vi "VIPM Project Parser_To String.vi"(11 "External Target Element":T1) -> (3 "Dependencies":string[](array[string]))   [LabVIEW 2019]
uses:
  Build/Project.Dependencies Finder.lvlibp/Ctl/Ctl_Dependency Element.ctl
  Build/Project.Dependencies Finder.lvlibp
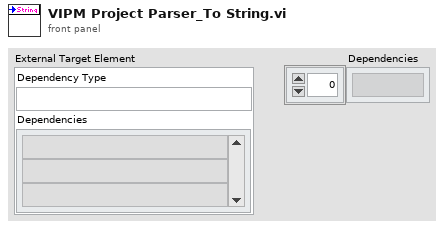
[diagram p1: front panel]
types:
  T1 = typedef "Project.Dependencies Finder.lvlibp/Ctl_Dependency Element.ctl" = cluster{"Dependency Type":string, "Dependencies":string[]}
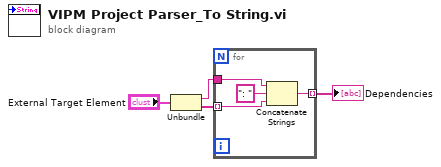
[diagram p0: block diagram]
diagram:
  n1 = Unbundle("External Target Element") -> ("Dependency Type"=w2:string, "Dependencies"=w3:string[])
  n2 = for {
    tunnel: w3 -> [w6] mode=indexing
    tunnel: w2 -> [w8]
    tunnel: [w5] -> w1 mode=indexing
    n3 = Concatenate Strings(w8, ": " ("string"), w6) -> (w5:string)
  }
  "Dependencies" <- w1
